vi "Loop RUS Sweep.vi"() -> ()   [LabVIEW 2010]
uses:
  RUS/Controls/Lock-in DAQ settings.ctl
  RUS/Controls/Sweep settings.ctl
  File/Controls/Save data settings.ctl
  File/Controls/File formats.ctl
panel:
  in  "short thermometer snapshot":T1={"ITC Temperature"=300.0, "ITC Set Temperature"=300.0, "LTC Temperature"=300.0, "LTC21 Address"="GPIB0::15::INSTR", "ITC503 Address"="GPIB0::24::INSTR"}
  in  "RUS loop":bool=TRUE
  in  "Stop RUS loop":bool
  in  "save frequency in":bool=TRUE
  out "log line":string="time=Oct24,2011__14:45:49\tLTC=35.35700\tITC=37.05000\t ITC_set=37.10000\t\t filename=35.35700K_1000_3000_102411.dat\t"
  out "writing log to":string="C:\\data\\RUS\\Experiment\\ProbeTest\\Probe8\\SrKIr0_1\\Sweep1\\Stability_102411.dat"
  in  "Save data settings":T2={"Save data"=TRUE, "Data Root Path"=path "C:/Data/RUS/system test/porous staff", "File Prefix"="", "File Format"=enum."ASCII", "Save column names"=TRUE, "File Comments"="<Description of the current file>", "User/Prj"="<User Name/Project Description>"}
  in  "Fast sweep settings":T4={"Update rate (Hz)"=180.0, "Start F, Hz"=400000.0, "Stop F"=2000000.0, "Number of points"=30000, "Amplitude"=2.1, "Init&amplitude"=TRUE, "IF"=1000.0, "Time constant"=0.003} {"IF" format="%#_6p"; "Amplitude" min=0.0 max=2.5; "Number of points" format="%.0p"; "Stop F" format="%#_6p"; "Start F, Hz" format="%#_6p"; "Update rate (Hz)" format="%0.2f"}
  out "minutes/sweep":dbl=2.7777777777777777
  out "kHz/second":dbl=9.600000000000001
  in  "Bypass error dialog":bool=TRUE
  in  "Lock-in DAQ settings":T5={"Lockin mode"=enum."NI-DAQ", "DAQmx Device"="Dev1", "SR Lockin"="GPIB0::10::INSTR", "Clock Multiplier"=64, "Low-pass filter"=enum."No filtering", "Ranges and couplings "=[{"Range"=2.5, "Coupling"=10106}], "Samples per read"=100, "Record IF"=TRUE, "Auto-phase"=TRUE} {"Ranges and couplings"."Coupling" items=["default"=-1, "RSE"=10083, "NRSE"=10078, "Differential"=10106, "Pseudodifferential"=12529]}
  in  "wait time between sweeps (min)":dbl
  in  "at end of every sweep":bool
  out "Global stop indicator":bool
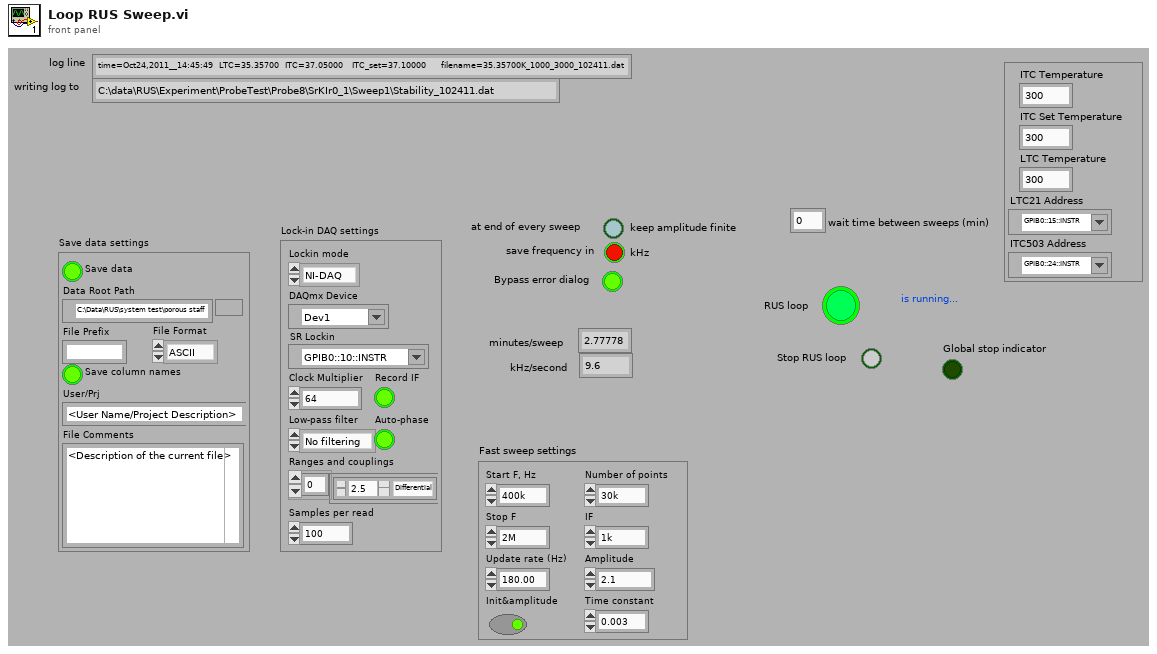
[diagram p1: front panel]
types:
  T1 = cluster{"ITC Temperature":dbl, "ITC Set Temperature":dbl, "LTC Temperature":dbl, "LTC21 Address":refnum<visa-resource-name>, "ITC503 Address":refnum<visa-resource-name>}
  T2 = typedef "Save data settings.ctl" = cluster{"Save data":bool, "Data Root Path":path, "File Prefix":string, "File Format":T3, "Save column names":bool, "File Comments":string, "User/Prj":string}
  T3 = typedef "File formats.ctl" = enum16{"TDMS", "ASCII", "BINARY"}
  T4 = typedef "Sweep settings.ctl" = cluster{"Update rate (Hz)":dbl, "Start F, Hz":dbl, "Stop F":dbl, "Number of points":i32, "Amplitude":dbl, "Init&amplitude":bool, "IF":dbl, "Time constant":dbl}
  T5 = typedef "Lock-in DAQ settings.ctl" = cluster{"Lockin mode":enum16{"SRS", "NI-DAQ"}, "DAQmx Device":tag, "SR Lockin":refnum<visa-resource-name>, "Clock Multiplier":i32, "Low-pass filter":enum16{"No filtering", "Butterworth", "Bessel"}, "Ranges and couplings ":cluster{"Range":dbl, "Coupling":i32}[], "Samples per read":i32, "Record IF":bool, "Auto-phase":bool}
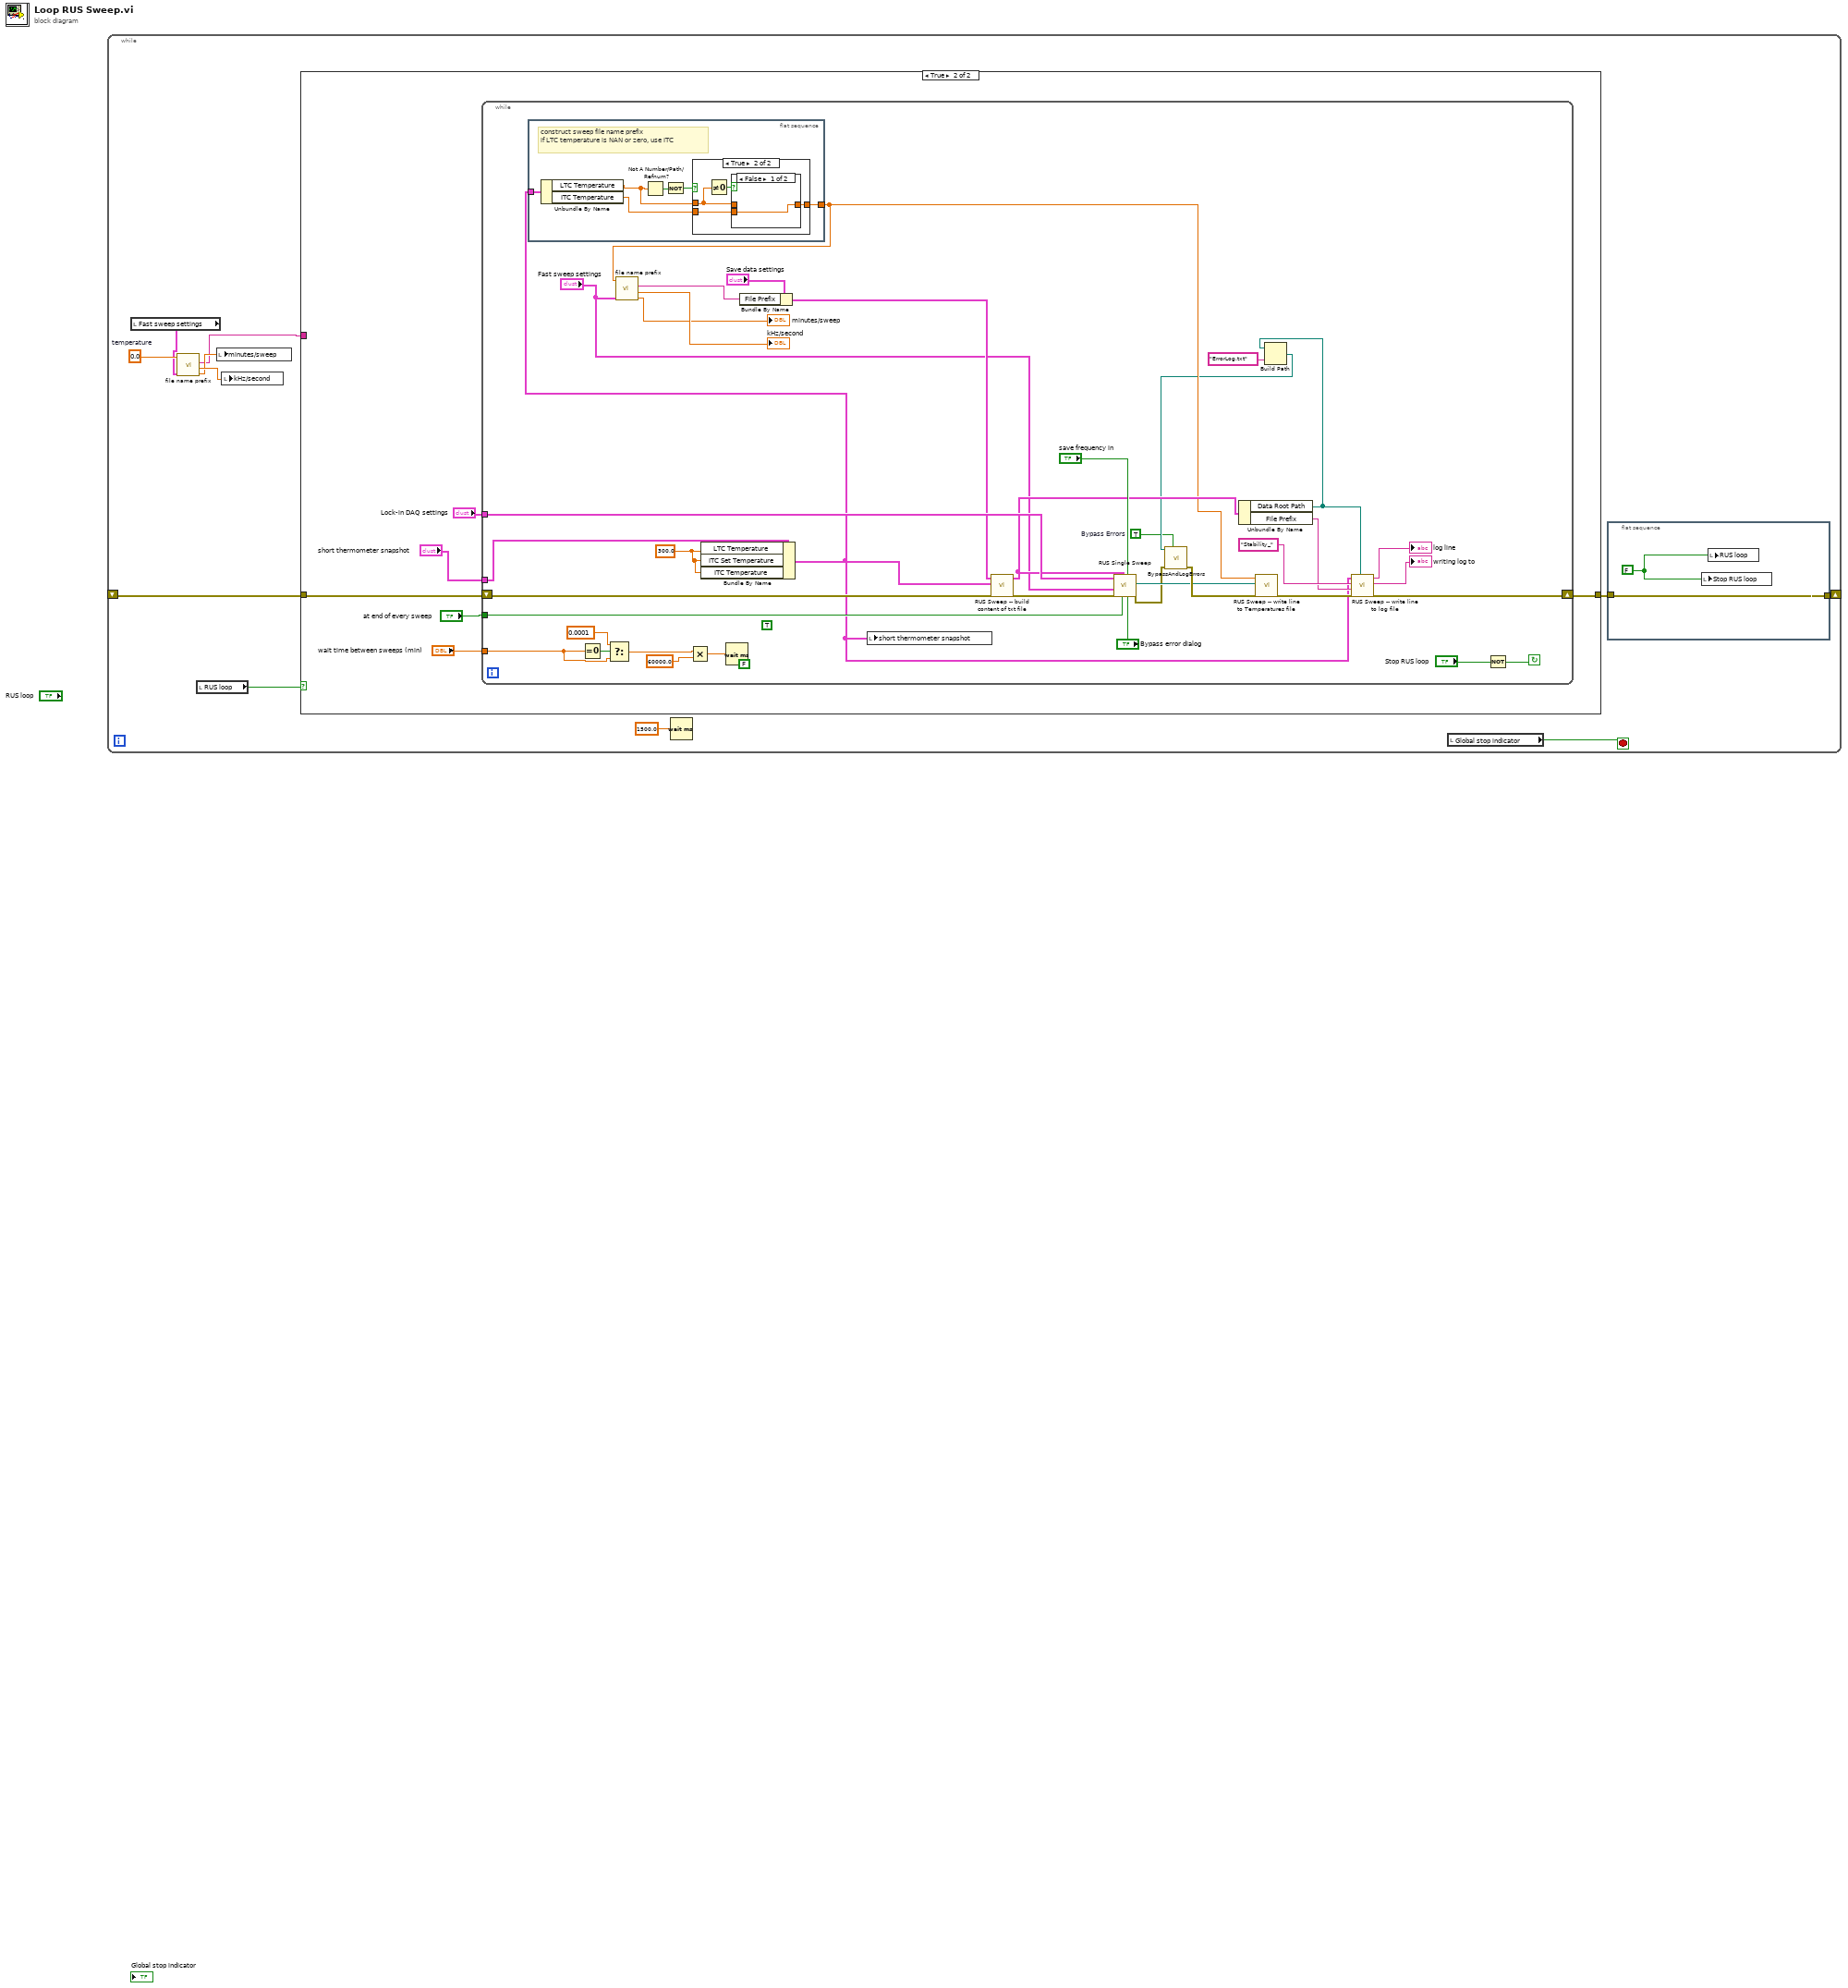
[diagram p0: block diagram]
diagram:
  n1 = while {
    shift-right: [w8] -> _
    shift-left: _ -> [w9]
    stop <- w11 stop-if-true
    w3 = 0.0  # temperature
    n2 = local read "Fast sweep settings"() -> (w2:T4)
    n3 = call "file name prefix.vi"("Fast sweep settings"=w2, "temperature"=w3) -> ("minutes/sweep"=w4:dbl, "kHz/second"=w5:dbl, "file name prefix"=w1:string)  [unwired: 7 in]
    n4 = local read "RUS loop"() -> (w10:bool)
    n5 = local write "minutes/sweep"(w4) -> ()
    n6 = local write "kHz/second"(w5) -> ()
    n7 = case shown="True" w10 {
      tunnel: [w14 w19] -> w7
      tunnel: w9 -> [w14 w18]
      tunnel: w1 -> [_ _]
      frame False {
      }
      frame True {
        n8 = while {
          tunnel: "at end of every sweep" -> [w58]
          tunnel: "Lock-in DAQ settings" -> [w57]
          tunnel: "short thermometer snapshot" -> [w25]
          shift-right: [w40] -> w19
          shift-left: w18 -> [w52]
          tunnel: "wait time between sweeps (min)" -> [w43]
          stop <- w30 continue-if-true
          w21 = TRUE  # Bypass Errors
          w29 = 300.0 ("ITC Temperature")
          (unwired) FALSE ("frequency  format")
          (unwired) TRUE ("set amplitude to zero \nat end of every sweep")
          n9 = flat-sequence {
            tunnel: [w60] -> w35
            tunnel: w24 -> [w64]
            frame #0 {
              # "construct sweep file name prefix\nif LTC temperature is NAN or zero, use ITC"
              n10 = Unbundle By Name(w64) -> ("LTC Temperature"=w61:dbl, "ITC Temperature"=w59:dbl)
              n11 = Not A Number/Path/Refnum?(number/path/refnum=w61) -> (NaN/Path/Refnum?=w63:bool)
              n12 = Not(x=w63) -> (.not. x?=w62:bool)
              n13 = case shown="True" w62 {
                tunnel: w61 -> [_ w67]
                tunnel: [w65 w68] -> w60
                tunnel: w59 -> [w65 w66]
                frame False {
                }
                frame True {
                  n14 = Not Equal To 0?(x=w67) -> (x != 0?=w69:bool)
                  n15 = case shown="False" w69 {
                    tunnel: [w70 w71] -> w68
                    tunnel: w67 -> [_ w71]
                    tunnel: w66 -> [w70 _]
                    frame False {
                    }
                    frame True {
                    }
                  }
                }
              }
            }
          }
          n16 = Equal To 0?(x=w43) -> (x = 0?=w45:bool)
          n17 = Select(t=0.0001, s=w45, f=w43) -> (s? t:f=w44:dbl)
          n18 = call "file name prefix.vi"("Fast sweep settings"="Fast sweep settings", "temperature"=w35) -> ("minutes/sweep"=→"minutes/sweep":dbl, "kHz/second"=→"kHz/second":dbl, "file name prefix"=w34:string)  [unwired: 7 in]
          n19 = Multiply(x=w44, y=60000.0) -> (x*y=w46:dbl)
          n20 = Bundle By Name(cluster=w25, "LTC Temperature"=w29, "ITC Set Temperature"=w29, "ITC Temperature"=w29) -> (w24:T1)
          n21 = Wait (ms)(milliseconds to wait=w46) -> ()  [unwired: 1 out]
          n22 = Bundle By Name(cluster="Save data settings", "File Prefix"=w34) -> (w39:T2)
          n23 = local write "short thermometer snapshot"(w24) -> ()
          n24 = call "RUS Sweep -- build content of txt file.vi"("error in"=w52, "thermometer snapshot"=w24, "Save data settings"=w39) -> ("error out"=w51:errorcluster, "Save data settings out"=w38:T2)  [unwired: 7 in]
          n25 = call "RUS Single Sweep.vi"("Bypass error dialog"="Bypass error dialog", "Divide something by something for Albert"="save frequency in", "Zero amplitude at the end"=w58, "Save data settings"=w38, "error in (no error)"=w51, "Fast swep settings"="Fast sweep settings", "Lock-in DAQ settings"=w57) -> ("error out"=w22:errorcluster, "Actual file path"=w48:path)  [unwired: 2 in, 1 out]
          n26 = Unbundle By Name(w38) -> ("Data Root Path"=w28:path, "File Prefix"=w37:string)
          n27 = Build Path(base path=w28, name or relative path="ErrorLog.txt") -> (appended path=w26:path)
          n28 = call "BypassAndLogErrors.vi"("Bypass Errors"=w21, "error in (no error)"=w22, "Log File Path"=w26) -> ("error out"=w50:errorcluster)  [unwired: 8 in]
          n29 = call "RUS Sweep -- write line to Temperatures file.vi"("error in"=w50, "Folder Path"=w48, "LTC Temperature"=w35) -> ("error out"=w49:errorcluster)  [unwired: 8 in]
          n30 = call "RUS Sweep -- write line to log file.vi"("base path"=w28, "error in (no error)"=w49, "current sweep file name"=w37, "base name"="Stability_", "thermometer snapshot"=w24) -> ("error out"=w40:errorcluster, "writing to"=→"writing log to":string, "log line"=→"log line":string)  [unwired: 4 in]
          n31 = Not(x="Stop RUS loop") -> (.not. x?=w30:bool)
        }
      }
    }
    n32 = Wait (ms)(milliseconds to wait=1500.0 ("y")) -> ()  [unwired: 1 out]
    n33 = local read "Global stop indicator"() -> (w11:bool)
    n34 = flat-sequence {
      tunnel: [w13] -> w8
      tunnel: w7 -> [w13]
      frame #0 {
        w12 = FALSE ("GO!")
        n35 = local write "Stop RUS loop"(w12) -> ()
        n36 = local write "RUS loop"(w12) -> ()
      }
    }
  }
